vi "Strafe Correction.vi"(6 "Steer":dbl, 9 "L Trigger":dbl, 10 "R Trigger":dbl, 11 "Max Steer":dbl) -> (0 "Angle":dbl, 2 "Gyro Steer":bool, 3 "Strafe Out":dbl)   [LabVIEW 2015]
uses:
  Common Code/Change Detect Boolean.vi
  Robot Global Data.vi
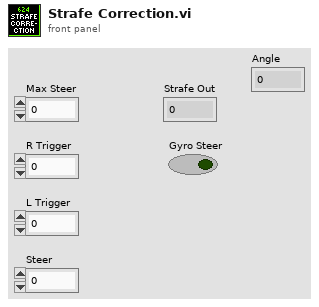
[diagram p1: front panel]
types:
  T1 = typedef "IMU Data.ctl" = cluster{"Pitch":sgl, "Roll":sgl, "Yaw":sgl, "Data Valid?":bool, "Temp":sgl, "MOVING":bool, "NAVX_CAL_STATUS":T2, "NAVX_OP_STATUS":T3, "YAW_STABLE":bool, "Accel X":sgl, "Accel Y":sgl, "Accel Z":sgl, "Accel Magnitude":sgl, "Pitch Rate":sgl, "Roll Rate":sgl, "Yaw Rate":sgl, "NavX Opened?":bool}
  T2 = typedef "navX-MXP IMU.lvlib/navX NAVX_CAL_STATUS.ctl" = u8
  T3 = typedef "navX-MXP IMU.lvlib/navX NAVX_OP_STATUS.ctl" = u8
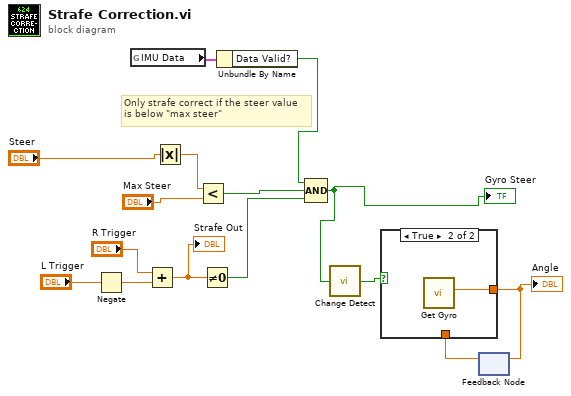
[diagram p0: block diagram]
diagram:
  # "Only strafe correct if the steer value\nis below \"max steer\""
  n1 = Negate(x="L Trigger") -> (-x=w11:dbl)
  n2 = global read "Robot Global Data.vi" "IMU Data"() -> (w2:T1)
  n3 = Add(x="R Trigger", y=w11) -> (x+y=w13:dbl)
  "Strafe Out" <- w13
  n4 = Absolute Value(x="Steer") -> (abs(x)=w4:dbl)
  n5 = Less?(x=w4, y="Max Steer") -> (x < y?=w14:bool)
  n6 = Not Equal To 0?(x=w13) -> (x != 0?=w15:bool)
  n7 = Unbundle By Name(w2) -> ("Data Valid?"=w1:bool)
  n8 = Compound Arithmetic op=AND(w1, w14, w15) -> (w6:bool)
  "Gyro Steer" <- w6
  n9 = call-poly "Change Detect.vi"("In"=w6) -> ("Changed?"=w9:bool)
  n10 = feedback #1() -> (w7:dbl)  [unwired: 1 in]
  n11 = case shown="True" w9 {
    tunnel: [w16 w17] -> w8
    tunnel: w7 -> [w16 _]
    frame False {
    }
    frame True {
      n12 = call "Get Gyro.vi"() -> ("Angle"=w17:dbl)  [unwired: 11 in]
    }
  }
  "Angle" <- w8
  n13 = feedback-in #1(w8) -> ()
